vi "go with sensor.vi"(0 "KNR in":T2, 1 "传感器类型":T1 items=["光感", "超声波"], 2 "方向":T1 items=["前进", "后退"], 3 "then go:":dbl, 11 "error in (no error)":errorcluster) -> (4 "KNR out":T2, 14 "offset":i32, 15 "error out":errorcluster)   [LabVIEW 2013]
uses:
  <userlib>/KNR OS 3.0 LabVIEW Toolkit/Type Definition/KNR3 Reference.ctl
  <userlib>/_FPGA Interface Advanced Tools/FPGA Interface Base/FPGA Interface Base.lvclass
  <userlib>/KNR OS 3.0 LabVIEW Toolkit/Type Definition/Resource.ctl
  <userlib>/KNR OS 3.0 LabVIEW Toolkit/Type Definition/DC Motor Port.ctl
  Global 1.vi
panel:
  in  "STOP 2":bool
  out "移动了":i32
  out "最后位置":i32
  out "右轮位置 4":i32
  out "左轮位置 4":i32
  out "右轮位置 3":i32
  out "左轮位置 3":i32
  in  "STOP 光感":bool
  out "光感读数":i32
  in  "STOP":bool
  out "超声波读数":i32
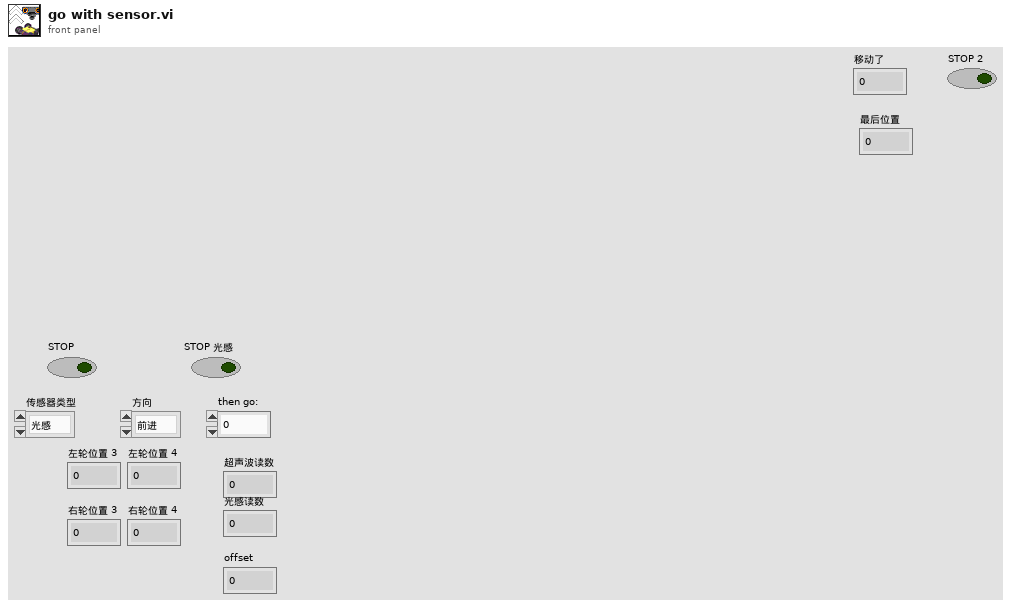
[diagram p1: front panel]
types:
  T1 = typedef "DC Motor Port.ctl" = u16
  T2 = typedef "KNR3 Reference.ctl" = cluster{"FPGA Session":refnum<class "FPGA Interface Base.lvclass">, "Resource":T3}
  T3 = typedef "Resource.ctl" = enum16{"KNRm_DDRC", "KNRm_DDDD", "KNRm_DDDR", "KNRm_DDDC", "KNR"}
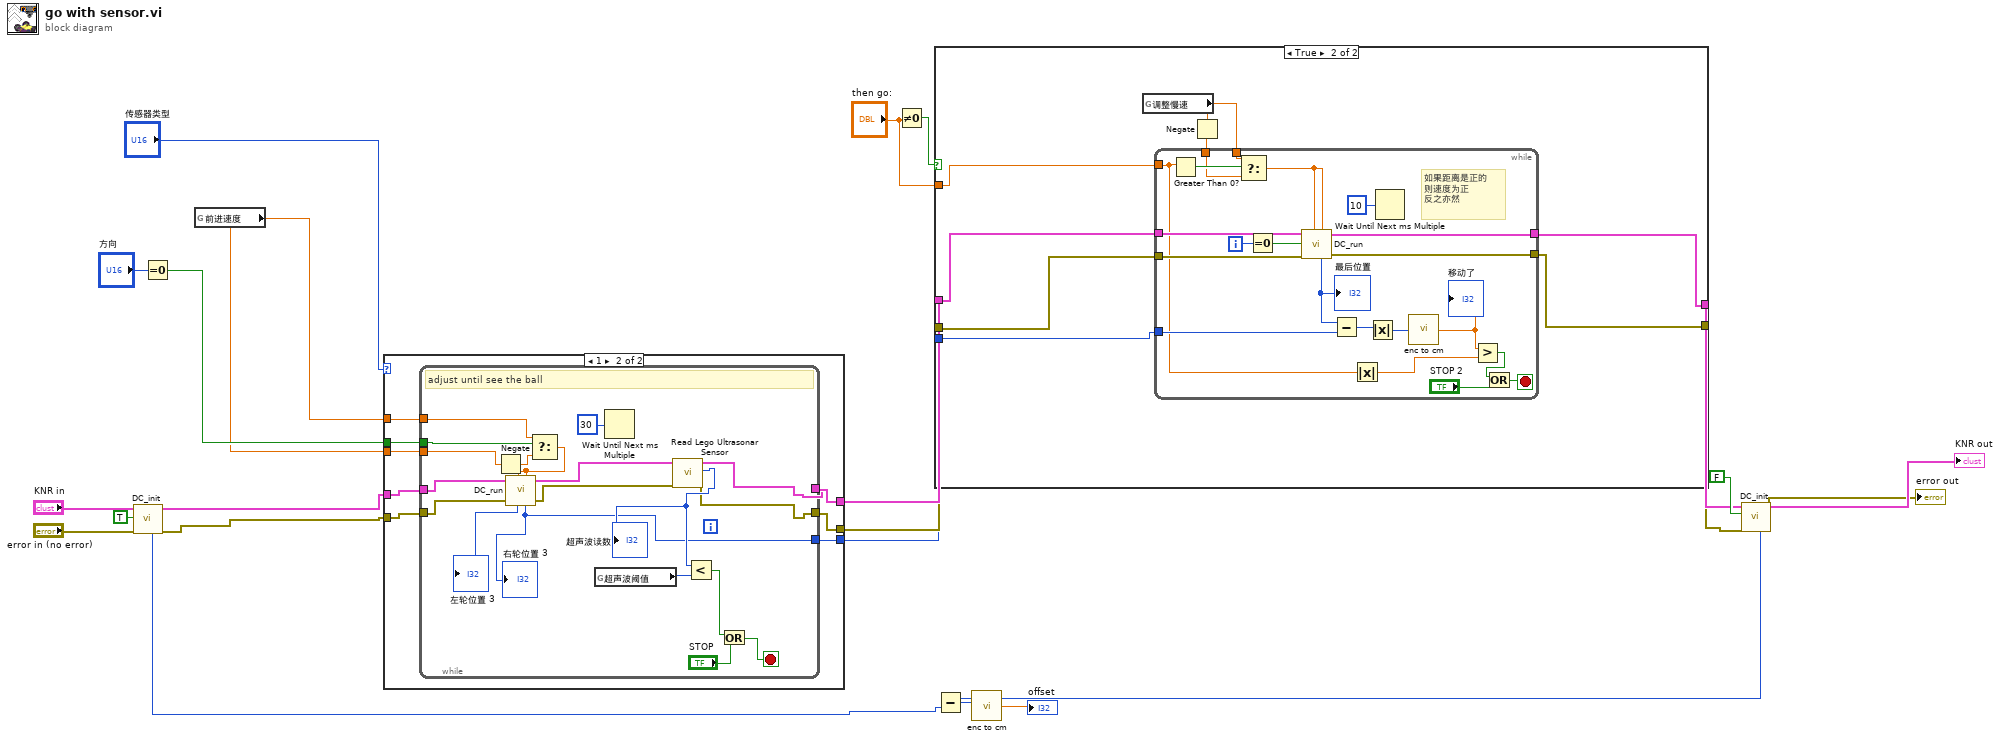
[diagram p0: block diagram]
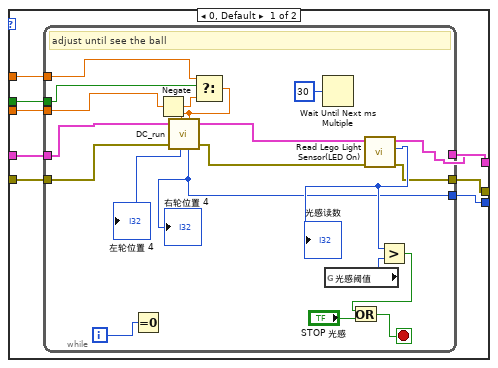
[diagram p3: hidden frame]
diagram:
  n1 = call "DC_init.vi"("error in (no error)"="error in (no error)", "Enable Motor(T)"=TRUE, "KNR in"="KNR in") -> ("error out"=w9:errorcluster, "KNR out"=w8:T2, "output\nposition 2"=w14:i32)  [unwired: 5 in, 1 out]
  n2 = Equal To 0?(x="方向") -> (x = 0?=w11:bool)
  n3 = global read "Global 1.vi" "前进速度"() -> (w10:dbl)
  n4 = case shown="1" "传感器类型" {
    tunnel: w8 -> [w31 w59]
    tunnel: w9 -> [w30 w58]
    tunnel: [w29 w57] -> w6
    tunnel: [w28 w56] -> w5
    tunnel: w10 -> [w25 w55]
    tunnel: w11 -> [w26 w54]
    tunnel: w10 -> [w27 w53]
    tunnel: [w24 w52] -> w1
    frame 0, Default {
      n5 = while {
        tunnel: w31 -> [w38]
        tunnel: w30 -> [w37]
        tunnel: [w44] -> w28
        tunnel: [w45] -> w29
        tunnel: w27 -> [w36]
        tunnel: w26 -> [w35]
        tunnel: w25 -> [w34]
        tunnel: [w32] -> w24
        i -> [w47]
        stop <- w51 stop-if-true
        # "adjust until see the ball"
        n6 = Equal To 0?(x=w47) -> ()  [unwired: 1 out]
        n7 = Negate(x=w34) -> (-x=w42:dbl)
        n8 = Select(t=w36, s=w35, f=w42) -> (s? t:f=w41:dbl)
        n9 = call "DC_run.vi"("KNR in"=w38, "speed_1"=w41, "error in (no error)"=w37, "speed_2"=w41) -> ("Position_1"=→"左轮位置 4":i32, "KNR out"=w40:T2, "Position_2"=w32:i32, "error out"=w39:errorcluster)  [unwired: 2 in]
        "右轮位置 4" <- w32
        n10 = Wait Until Next ms Multiple(millisecond multiple=u32 30) -> ()  [unwired: 1 out]
        n11 = global read "Global 1.vi" "光感阈值"() -> (w49:i32)
        n12 = call <userlib>:"Read Lego Light Sensor(LED On).vi"("error in (no error)"=w39, "KNR in"=w40) -> ("error out"=w44:errorcluster, "Row Value"=w46:u16, "KNR out"=w45:T2)  [unwired: 6 in, 1 out]
        "光感读数" <- w46
        n13 = Greater?(x=w46, y=w49) -> (0:w48:bool)
        n14 = Or(x=w48, y="STOP 光感") -> (x .or. y?=w51:bool)
      }
    }
    frame 1 {
      n15 = while {
        tunnel: w59 -> [w70]
        tunnel: w58 -> [w69]
        tunnel: [w73] -> w56
        tunnel: [w74] -> w57
        tunnel: w55 -> [w65]
        tunnel: w54 -> [w64]
        tunnel: w53 -> [w63]
        tunnel: [w60] -> w52
        stop <- w78 stop-if-true
        # "adjust until see the ball"
        n16 = Negate(x=w65) -> (-x=w66:dbl)
        n17 = Select(t=w63, s=w64, f=w66) -> (s? t:f=w62:dbl)
        n18 = call "DC_run.vi"("KNR in"=w70, "speed_1"=w62, "error in (no error)"=w69, "speed_2"=w62) -> ("Position_1"=→"左轮位置 3":i32, "KNR out"=w68:T2, "Position_2"=w60:i32, "error out"=w67:errorcluster)  [unwired: 2 in]
        "右轮位置 3" <- w60
        n19 = global read "Global 1.vi" "超声波阈值"() -> (w61:i32)
        n20 = Wait Until Next ms Multiple(millisecond multiple=u32 30) -> ()  [unwired: 1 out]
        n21 = call <userlib>:"Read Lego Ultrasonar Sensor.vi"("error in (no error)"=w67, "KNR in"=w68) -> ("error out"=w73:errorcluster, "distance(cm)"=w75:u8, "KNR out"=w74:T2)  [unwired: 7 in]
        "超声波读数" <- w75
        n22 = Less?(x=w75, y=w61) -> (x < y?=w76:bool)
        n23 = Or(x=w76, y="STOP") -> (x .or. y?=w78:bool)
      }
    }
  }
  n24 = Not Equal To 0?(x="then go:") -> (x != 0?=w7:bool)
  n25 = case shown="True" w7 {
    tunnel: w6 -> [w80 w86]
    tunnel: w5 -> [w79 w85]
    tunnel: [w80 w84] -> w4
    tunnel: [w79 w83] -> w3
    tunnel: "then go:" -> [_ w82]
    tunnel: w1 -> [_ w81]
    frame False {
    }
    frame True {
      n26 = global read "Global 1.vi" "调整慢速"() -> (w87:dbl)
      n27 = Negate(x=w87) -> (-x=w88:dbl)
      n28 = while {
        tunnel: w86 -> [w107]
        tunnel: w85 -> [w106]
        tunnel: [w98] -> w84
        tunnel: [w97] -> w83
        tunnel: w81 -> [w94]
        tunnel: w82 -> [w93]
        tunnel: w87 -> [w92]
        tunnel: w88 -> [w91]
        i -> [w103]
        stop <- w89 stop-if-true
        # "如果距离是正的\n则速度为正\n反之亦然"
        n29 = Greater Than 0?(x=w93) -> (x > 0?=w108:bool)
        n30 = Select(t=w92, s=w108, f=w91) -> (s? t:f=w105:dbl)
        n31 = Equal To 0?(x=w103) -> (x = 0?=w104:bool)
        n32 = call "DC_run.vi"("KNR in"=w107, "speed_1"=w105, "reinitialize? (F)"=w104, "error in (no error)"=w106, "speed_2"=w105) -> ("KNR out"=w98:T2, "Position_2"=w95:i32, "error out"=w97:errorcluster)  [unwired: 1 in, 1 out]
        "最后位置" <- w95
        n33 = Subtract(x=w95, y=w94) -> (x-y=w102:i32)
        n34 = Absolute Value(x=w93) -> (abs(x)=w101:dbl)
        n35 = Absolute Value(x=w102) -> (abs(x)=w99:i32)
        n36 = Wait Until Next ms Multiple(millisecond multiple=u32 10) -> ()  [unwired: 1 out]
        n37 = call "enc to cm.vi"("E"=w99) -> ("CM"=w96:dbl)  [unwired: 1 in]
        "移动了" <- w96
        n38 = Greater?(x=w96, y=w101) -> (0:w100:bool)
        n39 = Or(x=w100, y="STOP 2") -> (x .or. y?=w89:bool)
      }
    }
  }
  n40 = call "DC_init.vi"("error in (no error)"=w3, "Enable Motor(T)"=FALSE, "KNR in"=w4) -> ("error out"=→"error out":errorcluster, "KNR out"=→"KNR out":T2, "output\nposition 2"=w15:i32)  [unwired: 5 in, 1 out]
  n41 = Subtract(x=w15, y=w14) -> (x-y=w13:i32)
  n42 = call "enc to cm.vi"("E"=w13) -> ("CM"=→"offset":dbl)  [unwired: 1 in]
